vi "Wait for Operation Complete.vi"(8 "error in (no error)":errorcluster, 10 "Maximum Time (10000 ms)":i32=10000, 11 "VISA resource name":refnum<visa-resource-name>) -> (0 "error out":errorcluster, 3 "VISA resource name out":refnum<visa-resource-name>)   [LabVIEW 2012, in "Agilent PSG MXG Series.lvlib"]
doc: "Waits for the current operation to finish."
uses:
  <instrlib>/Agilent PSG MXG Series/Agilent PSG MXG Series.lvlib
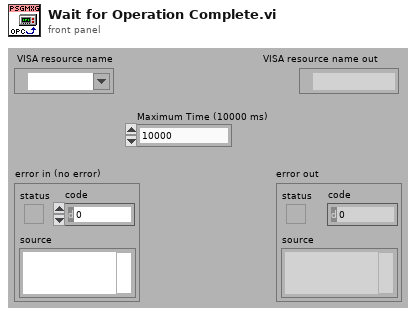
[diagram p1: front panel]
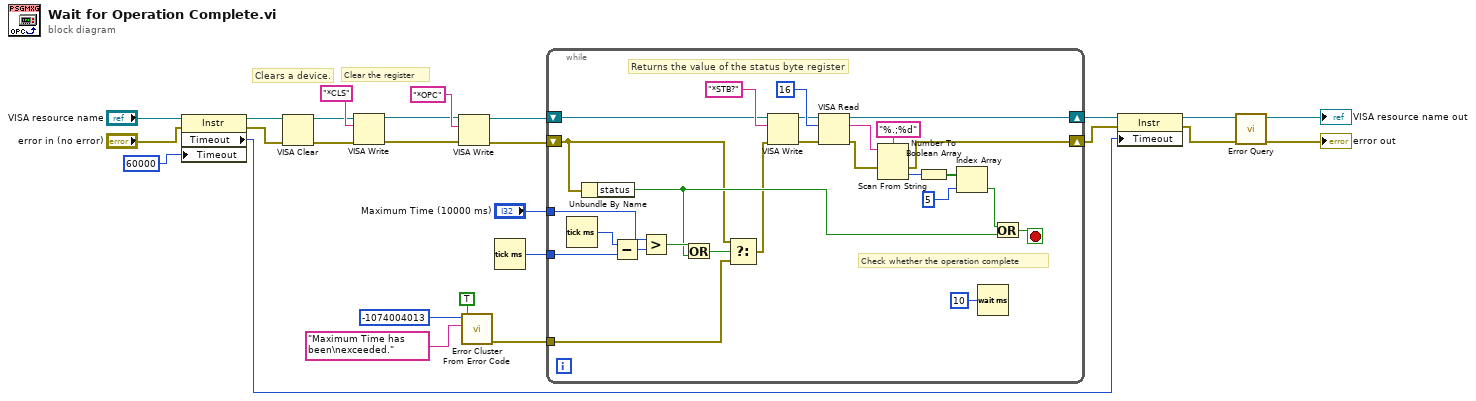
[diagram p0: block diagram]
diagram:
  # "Clears a device."
  # "Clear the register"
  n1 = property class="Instr"(reference="VISA resource name", error in="error in (no error)", "Timeout"=u32 60000 ("General Settings:Timeout Value")) -> (reference out=w12:refnum<visa-resource-name>, error out=w11:errorcluster, "Timeout"=w5:u32)
  n2 = VISA Clear(VISA resource name=w12, error in (no error)=w11) -> (VISA resource name out=w18:refnum<visa-resource-name>, error out=w17:errorcluster)
  n3 = VISA Write(VISA resource name=w18, write buffer="*CLS", error in (no error)=w17) -> (VISA resource name out=w16:refnum<visa-resource-name>, error out=w15:errorcluster)  [unwired: 1 out]
  n4 = VISA Write(VISA resource name=w16, write buffer="*OPC", error in (no error)=w15) -> (VISA resource name out=w13:refnum<visa-resource-name>, error out=w14:errorcluster)  [unwired: 1 out]
  n5 = call <vilib>:"Error Cluster From Error Code.vi"("show call chain? (False)"=TRUE, "error message (\"\")"="Maximum Time has been\nexceeded." ("error message (\"\")"), "error code (0)"=-1074004013) -> ("error out"=w20:errorcluster)  [unwired: 1 in, 5 out]
  n6 = Tick Count (ms)() -> (millisecond timer value=w25:u32)
  n7 = while {
    tunnel: "Maximum Time (10000 ms)" -> [w35]
    tunnel: w25 -> [w43]
    tunnel: w20 -> [w30]
    shift-right: [w41] -> w8
    shift-left: w14 -> [w28]
    shift-right: [w50] -> w9
    shift-left: w13 -> [w47]
    stop <- w36 stop-if-true
    # "Check whether the operation complete"
    # "Returns the value of the status byte register"
    n8 = Tick Count (ms)() -> (millisecond timer value=w44:u32)
    n9 = Unbundle By Name(w28) -> ("status"=w31:bool)
    n10 = Subtract(x=w44, y=w43) -> (x-y=w34:u32)
    n11 = Greater?(x=w35, y=w34) -> (0:w33:bool)
    n12 = Or(x=w33, y=w31) -> (x .or. y?=w32:bool)
    n13 = Select(t=w28, s=w32, f=w30) -> (s? t:f=w29:errorcluster)
    n14 = VISA Write(VISA resource name=w47, write buffer="*STB?", error in (no error)=w29) -> (VISA resource name out=w45:refnum<visa-resource-name>, error out=w46:errorcluster)  [unwired: 1 out]
    n15 = VISA Read(VISA resource name=w45, byte count=u32 16, error in (no error)=w46) -> (VISA resource name out=w50:refnum<visa-resource-name>, read buffer=w52:string, error out=w42:errorcluster)  [unwired: 1 out]
    n16 = Scan From String(format string="%.;%d", input string=w52, error in=w42) -> (error out=w41:errorcluster, output 1=w38:i32)  [unwired: 1 in, 3 out]
    n17 = Number To Boolean Array(number=w38) -> (Boolean array=w39:bool[])
    n18 = Index Array(array=w39, index=5) -> (element=w37:bool)
    n19 = Wait (ms)(milliseconds to wait=u32 10) -> ()  [unwired: 1 out]
    n20 = Or(x=w37, y=w31) -> (x .or. y?=w36:bool)
  }
  n21 = property class="Instr"(reference=w9, error in=w8, "Timeout"=w5) -> (reference out=w7:refnum<visa-resource-name>, error out=w6:errorcluster)
  n22 = call <instrlib>:"Error Query.vi"("error in (no error)"=w6, "VISA resource name"=w7) -> ("error out"=→"error out":errorcluster, "VISA resource name out"=→"VISA resource name out":refnum<visa-resource-name>)  [unwired: 8 out]
